vi "DSF.Engine.Memory.Cache.Plugin.Get Largest Count.All Types.vi"(8 "error in (no error)":errorcluster, 10 "Data Type Counts in":T1 {"U64" format="%d elements"; "U32" format="%d elements"; "U16" format="%d elements"; "U8" format="%d elements"; "I64" format="%d elements"; "I32" format="%d elements"; "I16" format="%d elements"; "I8" format="%d elements"; "DBL" format="%d elements"; "SGL" format="%d elements"; "Bool" format="%d elements"}, 11 "Plugin Cache in":refnum<class "DSF.Engine.Memory.Cache.Plugin.lvclass">) -> (0 "error out":errorcluster, 2 "Data Type Counts out":T1 {"U64" format="%d elements"; "U32" format="%d elements"; "U16" format="%d elements"; "U8" format="%d elements"; "I64" format="%d elements"; "I32" format="%d elements"; "I16" format="%d elements"; "I8" format="%d elements"; "DBL" format="%d elements"; "SGL" format="%d elements"; "Bool" format="%d elements"}, 3 "Plugin Cache out":refnum<class "DSF.Engine.Memory.Cache.Plugin.lvclass">)   [LabVIEW 2016, in "DSF.Engine.lvlib" / "DSF.Engine.Memory.Cache.Plugin.lvclass"]
uses:
  DSF.Engine.Memory.Cache.Plugin.lvclass
  Typedefs/DSF.Shared.Data Type Counts.ctl
  DSF.Engine.Memory.Cache.Plugin.lvclass/DSF.Engine.Memory.Cache.Plugin.ctl
  DSF.Engine.Memory.Cache.Transfer.lvclass/DSF.Engine.Memory.Cache.Transfer.ctl
  DSF.Engine.Memory.Cache.Transfer.Get Channel Configuration.vi
  DSF.Engine.Memory.Cache.Transfer.lvclass
  DSF.Shared.lvlib
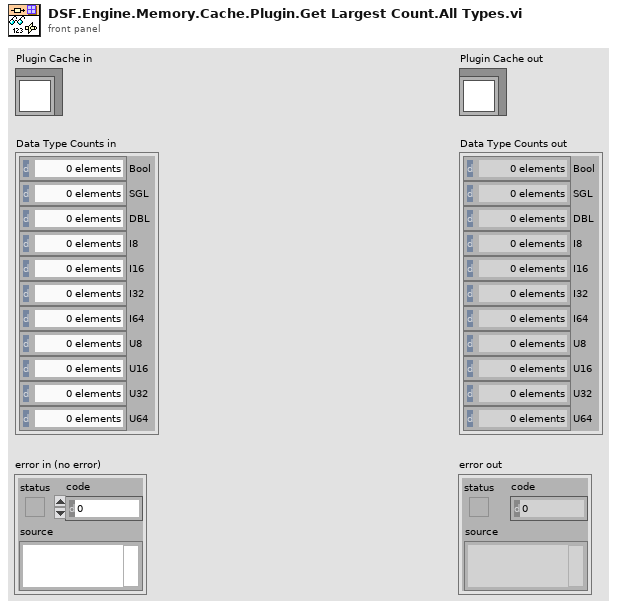
[diagram p1: front panel]
types:
  T1 = typedef "DSF.Shared.lvlib/DSF.Shared.Data Type Counts.ctl" = cluster{"Bool":u64, "SGL":u64, "DBL":u64, "I8":u64, "I16":u64, "I32":u64, "I64":u64, "U8":u64, "U16":u64, "U32":u64, "U64":u64}
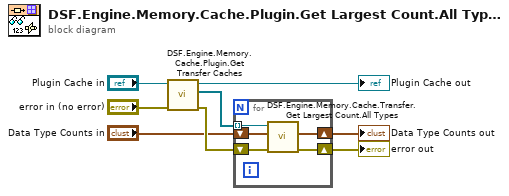
[diagram p0: block diagram]
diagram:
  n1 = call "DSF.Engine.Memory.Cache.Plugin.Get Transfer Caches.vi"("error in (no error)"="error in (no error)", "Plugin Cache in"="Plugin Cache in") -> ("error out"=w4:errorcluster, "Transfer Caches"=w6:refnum<class "DSF.Engine.Memory.Cache.Transfer.lvclass">[], "Plugin Cache out"=→"Plugin Cache out":refnum<class "DSF.Engine.Memory.Cache.Plugin.lvclass">)  [unwired: 7 in]
  n2 = for {
    shift-right: [w13] -> w1
    shift-left: "Data Type Counts in" -> [w12]
    tunnel: w6 -> [w11] mode=indexing
    shift-right: [w9] -> w3
    shift-left: w4 -> [w10]
    n3 = call "DSF.Engine.Memory.Cache.Transfer.Get Largest Count.All Types.vi"("error in (no error)"=w10, "Data Type Counts in"=w12, "Transfer Cache in"=w11) -> ("error out"=w9:errorcluster, "Data Type Counts out"=w13:T1)  [unwired: 6 in, 1 out]
  }
  "error out" <- w3
  "Data Type Counts out" <- w1
